vi "Create HH Page.vi"(8 "error in (no error)":errorcluster, 11 "Section Ptr":T1 format="%.0x") -> (0 "error out":errorcluster, 3 "Parent Ref out":T1 format="%.0x")   [LabVIEW 2015, in "DCM System Explorer.lvlib"]
uses:
  DCM System Explorer.lvlib
  <vilib>/NI Veristand/Custom Device API/Custom Device Item Ref.ctl
  Shared/DCM Constants and GUIDs.vi
  DCM Shared.lvlib
  <vilib>/NI VeriStand/Custom Device API/Custom Device API.lvlib
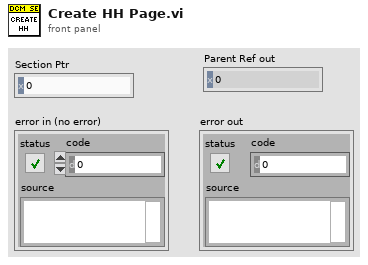
[diagram p1: front panel]
types:
  T1 = typedef "Custom Device API.lvlib/Custom Device Item Ref.ctl" = u64
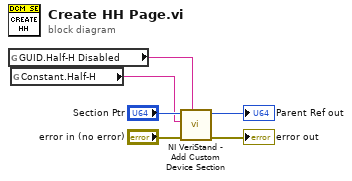
[diagram p0: block diagram]
diagram:
  n1 = global read "DCM Constants and GUIDs.vi" "GUID.Half-H Disabled"() -> (w4:string)
  n2 = global read "DCM Constants and GUIDs.vi" "Constant.Half-H"() -> (w3:string)
  n3 = call <vilib>:"NI VeriStand - Add Custom Device Section.vi"("GUID (Default Section)"=w4, "error in (no error)"="error in (no error)", "Section Name"=w3, "Parent Ref in"="Section Ptr") -> ("error out"=→"error out":errorcluster, "Parent Ref out"=→"Parent Ref out":T1)  [unwired: 4 in, 2 out]
